vi "Remove Header Bytes.vi"(2 "Bytes/Msg with header":u64) -> (4 "Bytes/Msg without header":u64)   [LabVIEW 2021, in "ChannelCommon.lvlib"]
uses:
  ChannelCommon.lvlib
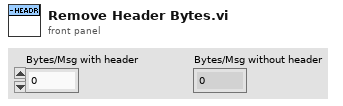
[diagram p1: front panel]
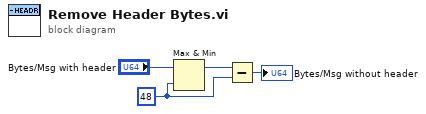
[diagram p0: block diagram]
diagram:
  w1 = u64 48 ("value")
  n1 = Max & Min(x="Bytes/Msg with header", y=w1) -> (max(x,y)=w3:u64)  [unwired: 1 out]
  n2 = Subtract(x=w3, y=w1) -> (x-y=→"Bytes/Msg without header":u64)
